vi "lookfordata.vi"(1 "Header":string, 2 "string":string) -> (0 "output string":string)   [LabVIEW 2011]
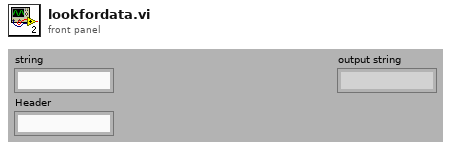
[diagram p1: front panel]
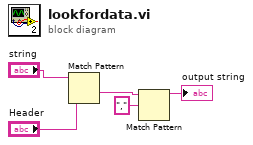
[diagram p0: block diagram]
diagram:
  n1 = Match Pattern(string="string", regular expression="Header") -> (after substring=w1:string)  [unwired: 4 out]
  n2 = Match Pattern(string=w1, regular expression=",") -> (before substring=→"output string":string)  [unwired: 4 out]
